vi "Constructor by Table Config.vi"(8 "error in (no error)":errorcluster, 9 "Field Factory Type":refnum<class "Column Factory.lvclass">, 10 "Table Configuration":refnum<class "Table Configuration Interface.lvclass">, 11 "Form from Table Configuration in":refnum<class "Form from Table Configuration.lvclass">) -> (0 "error out":errorcluster, 3 "Form from Table Configuration out":refnum<class "Form from Table Configuration.lvclass">)   [LabVIEW 2020, in "Panel Form Controller.lvlib" / "Form from Table Configuration.lvclass"]
uses:
  Form from Table Configuration.lvclass
  C:/Users/User/Desktop/Raman Program/Database OOP/source/Forms AF/Forms Controller/Configuration/Controller Configuration/Panel Form Controller Configuration.lvclass
  Database OOP/Table Libraries/Table Configuration Interface/Table Configuration Interface.lvclass
  Database OOP/Column Libraries/Basic Columns/Column Configuration/Column Factory Parent Class/Column Factory.lvclass
  Form from Table Configuration.lvclass/Form from Table Configuration.ctl
  Controller Configuration/Panel Form Controller Configuration.lvclass/Panel Form Controller Configuration.ctl
  Controller Configuration/Panel Form Controller Configuration.lvclass
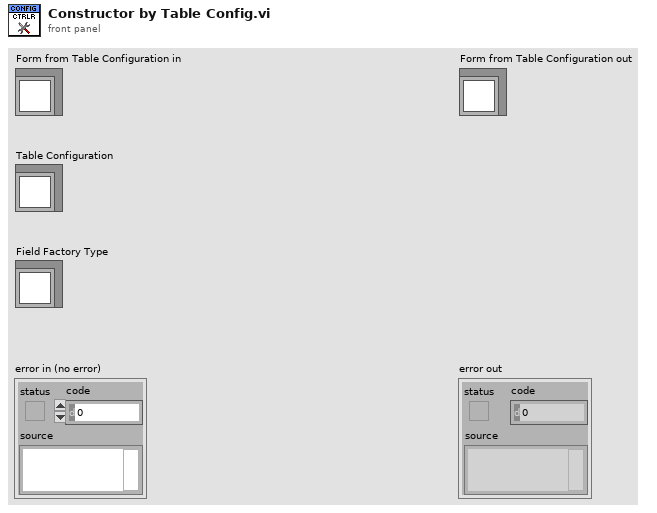
[diagram p1: front panel]
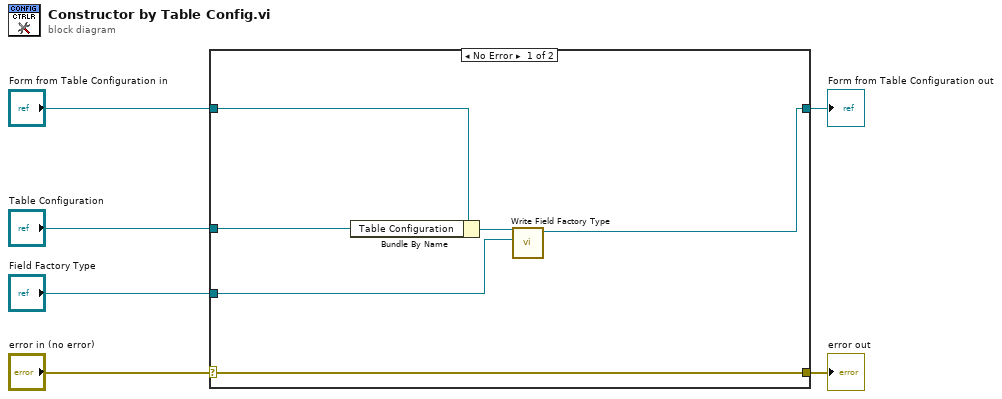
[diagram p0: block diagram]
diagram:
  n1 = case shown="No Error" "error in (no error)" {
    selector: "error in (no error)" -> [w12 w14]
    tunnel: [w12 w14] -> w5
    tunnel: [w7 w13] -> w3
    tunnel: "Form from Table Configuration in" -> [w11 w13]
    tunnel: "Table Configuration" -> [w10 _]
    tunnel: "Field Factory Type" -> [w8 _]
    frame No Error {
      n2 = Bundle By Name(cluster=w11, "Table Configuration"=w10) -> (w9:refnum<class "Form from Table Configuration.lvclass">)
      n3 = call "Write Field Factory Type.vi"("Field Factory Type"=w8, "Panel Form Controller Configuration in"=w9) -> ("Panel Form Controller Configuration out"=w7:refnum<class "Form from Table Configuration.lvclass">)  [unwired: 8 in, 1 out]
    }
    frame Error {
    }
  }
  "error out" <- w5
  "Form from Table Configuration out" <- w3
